vi "rotate_calculate_2.vi"(10 "pieceOfWorld":T2[][](array[typedef]), 11 "input cluster":T1) -> (1 "angle":dbl, 2 "full round":bool, 3 "output cluster":T1)   [LabVIEW 2015, in "PolyVIEW.lvclass"]
uses:
  PolyVIEW.lvclass
  actors/world/typedefs/worldCell_cluster.ctl
  actors/world/typedefs/markValue_cluster.ctl
  actors/world/typedefs/markValue.ctl
  actors/world/typedefs/markVolume.ctl
  actors/world/typedefs/amountOfFood.ctl
  actors/world/typedefs/anthillType_enum.ctl
  Memory.ctl
  actors/world/world.lvlib
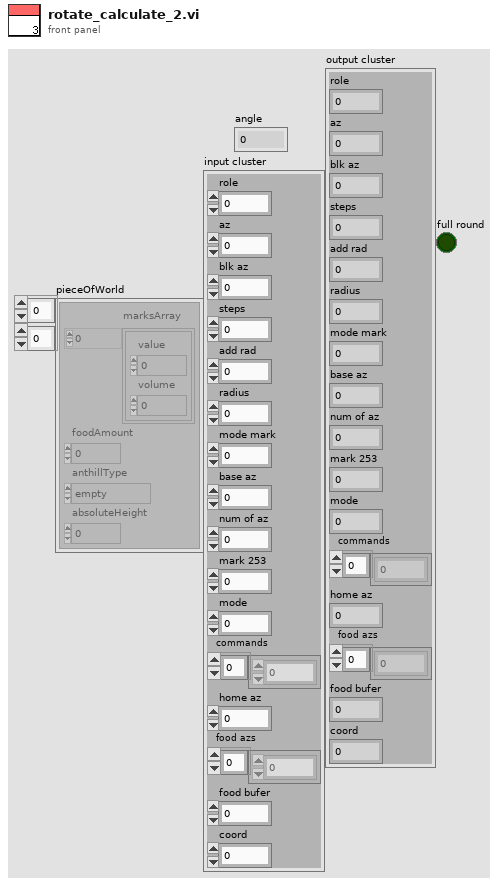
[diagram p1: front panel]
types:
  T1 = typedef "PolyVIEW.lvclass/Memory.ctl" = cluster{"role":i32, "az":i32, "blk az":i32, "steps":dbl, "add rad":i32, "radius":dbl, "mode mark":u32, "base az":dbl, "num of az":u32, "mark 253":u32, "mode":u32, "commands":i32[], "home az":dbl, "food azs":dbl[], "food bufer":dbl, "coord":cdb}
  T2 = typedef "world.lvlib/worldCell_cluster.ctl" = cluster{"marksArray":T3[], "foodAmount":T6, "anthillType":T7, "absoluteHeight":u8}
  T3 = typedef "world.lvlib/markValue_cluster.ctl" = cluster{"value":T4, "volume":T5}
  T4 = typedef "world.lvlib/markValue.ctl" = u8
  T5 = typedef "world.lvlib/markVolume.ctl" = u16
  T6 = typedef "world.lvlib/amountOfFood.ctl" = i32
  T7 = typedef "world.lvlib/anthillType_enum.ctl" = enum16{"empty", "own", "rival"}
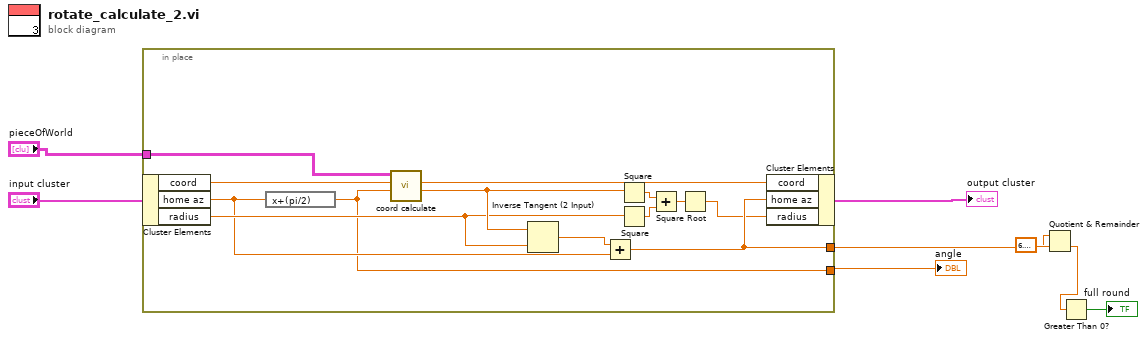
[diagram p0: block diagram]
diagram:
  n1 = in-place {
    in-place-border: "pieceOfWorld" -> [w21]
    in-place-border: [w9] -> w5
    in-place-border: [w14] -> w4
    n2 = in-place-cluster #1("input cluster") -> ("coord"=w15:cdb, "home az"=w10:dbl, "radius"=w12:dbl)
    n3 = expression code="x+(pi/2)"(w10) -> (w9:dbl)
    n4 = call "coord calculate.vi"("theta"=w9, "coord in"=w15, "pieceOfWorld in"=w21) -> ("length"=w18:dbl, "coord out"=w13:cdb)  [unwired: 7 in]
    n5 = Inverse Tangent (2 Input)(1:w12, 2:w18) -> (0:w20:dbl)
    n6 = Add(x=w20, y=w10) -> (x+y=w14:dbl)
    n7 = Square(x=w18) -> (x^2=w16:dbl)
    n8 = Square(x=w12) -> (x^2=w17:dbl)
    n9 = Add(x=w16, y=w17) -> (x+y=w19:dbl)
    n10 = Square Root(x=w19) -> (sqrt(x)=w11:dbl)
    n11 = in-place-cluster #1("coord"=w13, "home az"=w14, "radius"=w11) -> (→"output cluster":T1)
  }
  "angle" <- w5
  n12 = Quotient & Remainder(x=w4, y=6.283185307179586) -> (floor(x/y)=w7:dbl)  [unwired: 1 out]
  n13 = Greater Than 0?(x=w7) -> (x > 0?=→"full round":bool)
